vi "Reply Loop.vi"(8 "error in (no error)":errorcluster, 11 "Mock Sift Proxy Server in":refnum<class "Mock Sift Proxy Server.lvclass">) -> (0 "error out":errorcluster, 3 "Mock Sift Proxy Server out":refnum<class "Mock Sift Proxy Server.lvclass">)   [LabVIEW 2024, in "Mock Sift Proxy Server.lvclass"]
uses:
  Mock Sift Proxy Server.lvclass
  Private/Typedefs/Messages/JSON Response.ctl
  Mock Sift Proxy Server.lvclass/Mock Sift Proxy Server.ctl
  <vilib>/ErrorRing/Error Ring.xnode
  <vilib>/addons/_JKI.lib/Serialization/JSON/JKI JSON Serialization.lvlib
  Sift Client.lvlib
panel:
  out "data out":string
  in  "JSON Response":T1
  out "data in":string
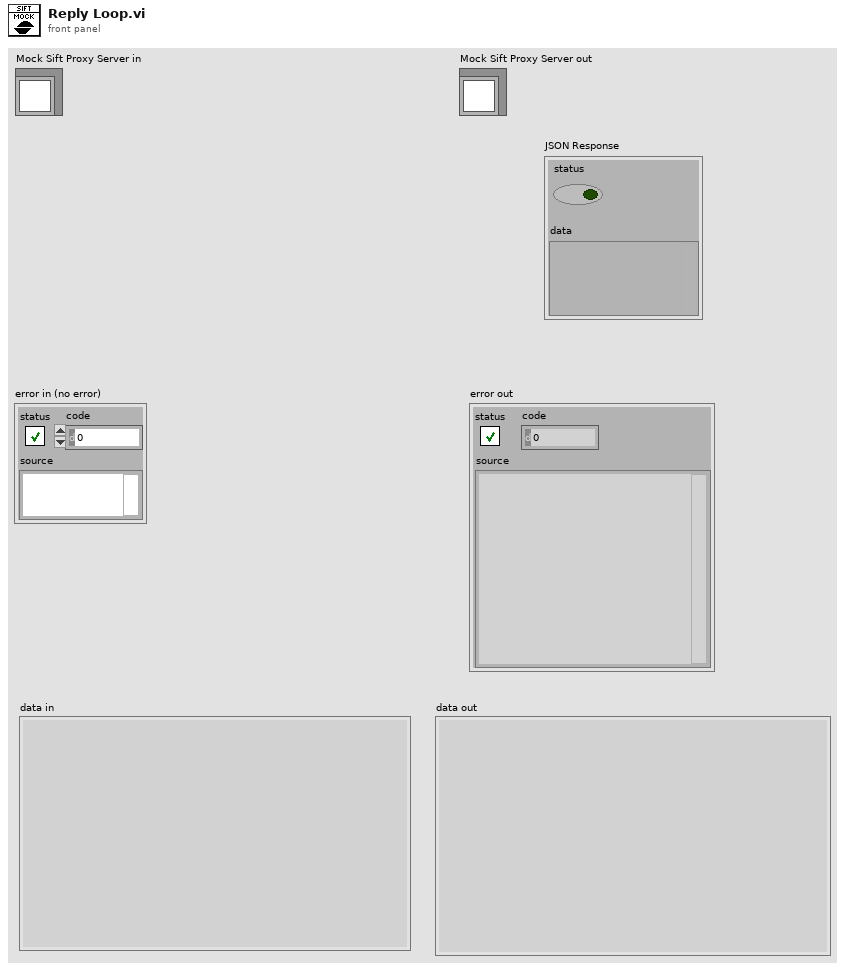
[diagram p1: front panel]
types:
  T1 = typedef "Sift Client.lvlib/JSON Response.ctl" = cluster{"status":bool, "data":variant}
  T2 = enum16{"Standard", "Buffered", "CRLF", "Immediate"}
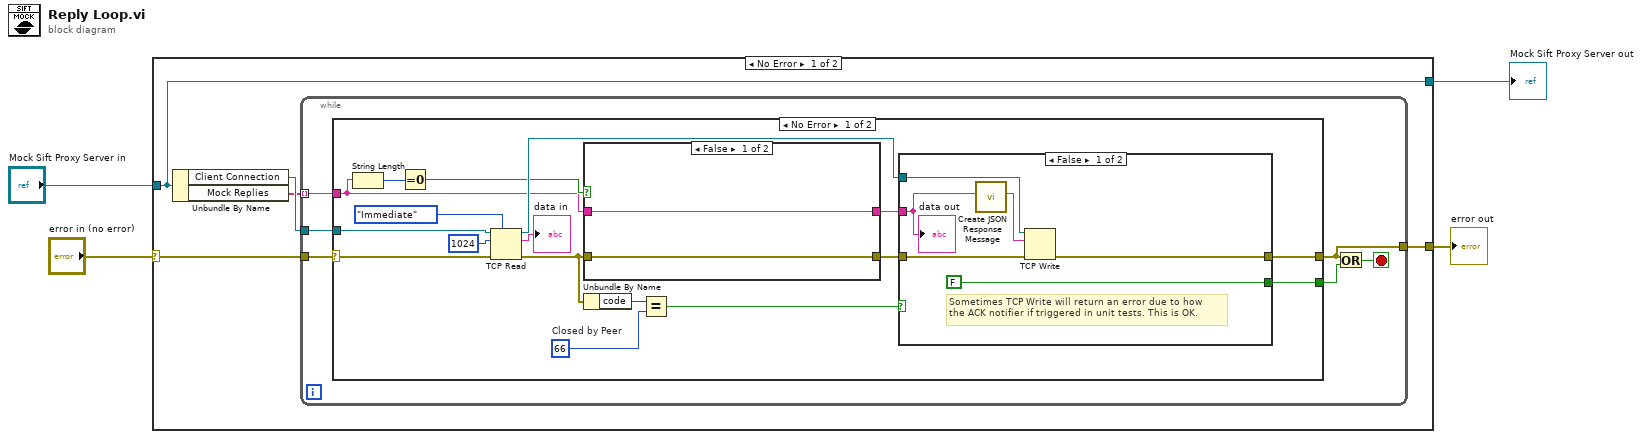
[diagram p0: block diagram]
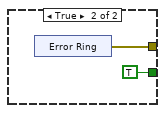
[diagram p2: hidden frame]
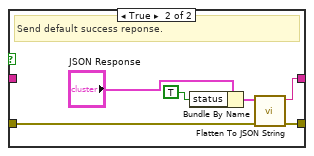
[diagram p3: hidden frame]
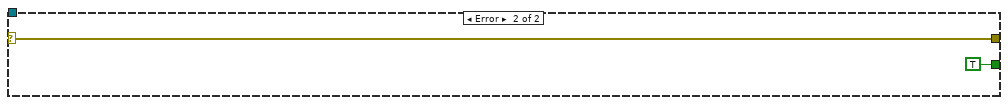
[diagram p4: hidden frame]
diagram:
  n1 = case shown="No Error" "error in (no error)" {
    selector: "error in (no error)" -> [w6 w53]
    tunnel: [w5 w53] -> w3
    tunnel: [w9 w52] -> w1
    tunnel: "Mock Sift Proxy Server in" -> [w9 w52]
    frame No Error {
      n2 = Unbundle By Name(w9) -> ("Client Connection"=w8:refnum<k5>, "Mock Replies"=w7:string[])
      n3 = while {
        tunnel: w8 -> [w15]
        tunnel: w7 -> [w14] mode=indexing
        tunnel: w6 -> [w13]
        tunnel: [w11] -> w5
        stop <- w12 stop-if-true
        n4 = case shown="No Error" w13 {
          selector: w13 -> [w19 w51]
          tunnel: w15 -> [w32 _]
          tunnel: [w29 w51] -> w11
          tunnel: w14 -> [w18 _]
          tunnel: [w20 TRUE] -> w10
          frame No Error {
            w22 = 66  # Closed by Peer
            n5 = String Length(string=w18) -> (length=w30:i32)
            n6 = Equal To 0?(x=w30) -> (x = 0?=w27:bool)
            n7 = TCP Read(connection ID=w32, bytes to read=1024, error in (no error)=w19, 7:T2."Immediate" ("mode (standard)")) -> (connection ID out=w31:refnum<k5>, data out=→"data in":string, error out=w17:errorcluster)  [unwired: 1 in]
            n8 = case shown="False" w27 {
              tunnel: [w43 w46] -> w28
              tunnel: w18 -> [w43 _]
              tunnel: w17 -> [w42 w45]
              tunnel: [w42 w44] -> w16
              frame False {
              }
              frame True {
                # "Send default success reponse."
                n9 = Bundle By Name(cluster="JSON Response", "status"=TRUE) -> (w47:T1)
                n10 = call <vilib>:"Flatten To JSON String.vi"("error in"=w45, "Variant"=w47) -> ("error out"=w44:errorcluster, "JSON String"=w46:string)  [unwired: 8 in]
              }
            }
            n11 = Unbundle By Name(w17) -> ("code"=w23:i32)
            n12 = Equal?(x=w23, y=w22) -> (x = y?=w21:bool)
            n13 = case shown="False" w21 {
              tunnel: w31 -> [w38 _]
              tunnel: [w37 w39] -> w29
              tunnel: w28 -> [w34 _]
              tunnel: [FALSE TRUE] -> w20
              tunnel: w16 -> [w35 _]
              frame False {
                # "Sometimes TCP Write will return an error due to how\nthe ACK notifier if triggered in unit tests. This is OK."
                n14 = call "Create JSON Response Message.vi"("Data"=w34) -> ("Message"=w33:string)  [unwired: 10 in]
                n15 = TCP Write(connection ID=w38, data in=w33, error in (no error)=w35) -> (error out=w37:errorcluster)  [unwired: 1 in, 2 out]
                "data out" <- w34
              }
              frame True {
                n16 = xnode "Error Ring"() -> ("error out"=w39:errorcluster)
              }
            }
          }
          frame Error {
          }
        }
        n17 = Or(x=w11, y=w10) -> (x .or. y?=w12:bool)
      }
    }
    frame Error {
    }
  }
  "error out" <- w3
  "Mock Sift Proxy Server out" <- w1
